vi "ITC503 Init.vi"(1 "ITC Selector":refnum<vi>) -> ()   [LabVIEW 2010]
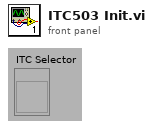
[diagram p1: front panel]
types:
  T1 = typedef "ITCSetupArray.ctl" = T2[]
  T2 = typedef "ITCSetup.ctl" = cluster{"Description":string, "IO Info":T3}
  T3 = typedef "ITCIO.ctl" = cluster{"Address":T4, "Version":T5, "Ch 1 dec places":i16, "Ch 2 dec places":i16, "Ch 3 dec places":i16, "Ch1 Name":string, "Ch2 Name":string, "Ch3 Name":string}
  T4 = typedef "OxfordAddress.ctl" = cluster{"Com Port":i32, "ISOBUS Address":i32, "GPIB Address":i16, "Communication":enum16{"RS232", "ISOBUS", "GPIB", "Gateway"}}
  T5 = typedef "ITCVersion.ctl" = enum16{"ITC502", "ITC503", "ITC601"}
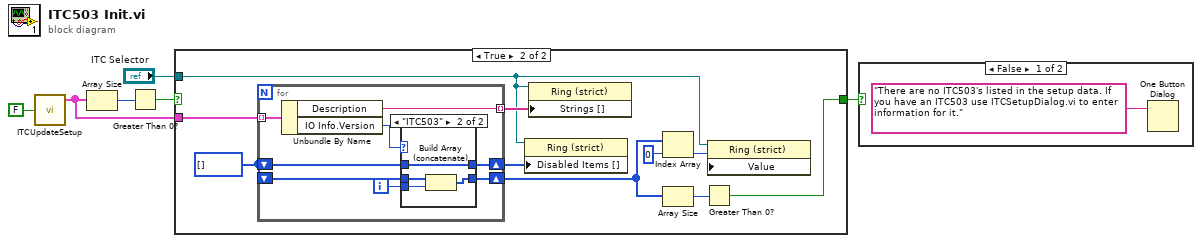
[diagram p0: block diagram]
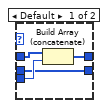
[diagram p3: hidden frame]
diagram:
  n1 = call "ITCUpdateSetup.vi"("Write to disk?"=FALSE) -> ("ITC Setup(read)"=w3:T1)  [unwired: 3 in, 1 out]
  n2 = Array Size(array=w3) -> (size(s)=w4:i32)
  n3 = Greater Than 0?(x=w4) -> (x > 0?=w5:bool)
  n4 = case shown="True" w5 {
    selector: w5 -> [w7 _]
    tunnel: w3 -> [_ w17]
    tunnel: [w7 w9] -> w6
    tunnel: "ITC Selector" -> [_ w8]
    frame False {
    }
    frame True {
      w14 = i32[] [] ("Array Constant")
      n5 = for {
        tunnel: [w25] -> w16 mode=indexing
        tunnel: w17 -> [w24] mode=indexing
        shift-right: [w21] -> w15
        shift-left: w14 -> [w22]
        shift-right: [w18] -> w11
        shift-left: w14 -> [w19]
        i -> [w20]
        n6 = Unbundle By Name(w24) -> ("Description"=w25:string, "IO Info.Version"=w23:T5)
        n7 = case shown="\"ITC503\"" w23 {
          tunnel: w22 -> [w27 w33]
          tunnel: [w29 w33] -> w21
          tunnel: w20 -> [w28 w31]
          tunnel: w19 -> [w26 w32]
          tunnel: [w26 w30] -> w18
          frame Default {
            n8 = Build Array (concatenate)(w27, w28) -> (w29:i32[])
          }
          frame "ITC503" {
            n9 = Build Array (concatenate)(w32, w31) -> (w30:i32[])
          }
        }
      }
      n10 = property on="Eigenschaftsknoten" class="Ring (strict)"(reference=w8, "Disabled Items []"=w15) -> ()  [unwired: 1 in, 2 out]
      n11 = property on="Eigenschaftsknoten" class="Ring (strict)"(reference=w8, "Strings []"=w16) -> ()  [unwired: 1 in, 2 out]
      n12 = Index Array(array=w11, index=0 ("Index")) -> (element=w12:i32)
      n13 = Array Size(array=w11) -> (size(s)=w10:i32)
      n14 = Greater Than 0?(x=w10) -> (x > 0?=w9:bool)
      n15 = property class="Ring (strict)"(reference=w8, "Value"=w12) -> ()  [unwired: 1 in, 2 out]
    }
  }
  n16 = case shown="False" w6 {
    frame False {
      n17 = One Button Dialog(message="There are no ITC503's listed in the setup data. If you have an ITC503 use ITCSetupDialog.vi to enter information for it.") -> ()  [unwired: 1 in, 1 out]
    }
    frame True {
    }
  }
